vi "Single-Point Tracking.vi"() -> ()   [LabVIEW 2021]
uses:
  <vilib>/myRIO/Instrument Drivers/Onboard IO/I2C/typedefs/I2C User Configuration.ctl
  <vilib>/myRIO/Instrument Drivers/Onboard IO/I2C/typedefs/I2C Transfer Rate.ctl
  <vilib>/myRIO/Instrument Drivers/Onboard IO/I2C/typedefs/I2C Reference.ctl
  <vilib>/myRIO/Common/Instrument Driver Framework/Utilities/typedefs/myRIO Generic Hardware Reference.ctl
  <vilib>/myRIO/Common/Instrument Driver Framework/Utilities/typedefs/Hardware Version Enum.ctl
  <vilib>/myRIO/Common/Instrument Driver Framework/Utilities/typedefs/myRIO v1.0 Reference.ctl
  <vilib>/myRIO/Common/Instrument Driver Framework/Utilities/typedefs/Generic FPGA Reference.ctl
  <vilib>/myRIO/Common/Instrument Driver Framework/myRIO v1.0/I2C/typedefs/I2C Channels Enum.ctl
  <vilib>/myRIO/Instrument Drivers/Onboard IO/I2C/typedefs/I2C Configuration.ctl
  <vilib>/userDefined/High Color/nirio_resource_hc.ctl
  <vilib>/myRIO/Instrument Drivers/Onboard IO/DIO/typedefs/DIO Reference.ctl
  <vilib>/myRIO/Common/Instrument Driver Framework/myRIO v1.0/DIO/typedefs/DIO Channels List.ctl
  <vilib>/myRIO/Common/Instrument Driver Framework/myRIO v1.0/DIO/typedefs/DIO Channels Enum.ctl
  <vilib>/myRIO/Instrument Drivers/Onboard IO/PWM/typedefs/PWM Reference.ctl
  <vilib>/myRIO/Common/Instrument Driver Framework/myRIO v1.0/PWM/typedefs/PWM Channels Enum.ctl
  <vilib>/myRIO/Instrument Drivers/Onboard IO/PWM/typedefs/PWM Configuration.ctl
  <vilib>/myRIO/Common/Instrument Driver Framework/Utilities/vis/Is FPGA Ref Available.vi
  <vilib>/myRIO/Common/Instrument Driver Framework/myRIO v1.0/I2C/vis/myRIO v1.1 Open I2C.vi
  <vilib>/myRIO/Instrument Drivers/Onboard IO/I2C/vis/Configure.vi
  <vilib>/myRIO/Instrument Drivers/Onboard IO/I2C/vis/Write.vi
  <vilib>/myRIO/Common/Instrument Driver Framework/myRIO v1.0/PWM/vis/myRIO v1.1 Open PWM.vi
  <vilib>/myRIO/Instrument Drivers/Onboard IO/PWM/vis/Set Duty Cycle and Frequency.vi
  <vilib>/myRIO/Common/Instrument Driver Framework/myRIO v1.0/DIO/vis/myRIO v1.1 Open DIO.vi
  <vilib>/myRIO/Instrument Drivers/Onboard IO/DIO/vis/Write.vi
  <vilib>/myRIO/Instrument Drivers/Onboard IO/I2C/vis/Write Read.vi
  <vilib>/Analysis/baseanly.llb/Mean (DBL).vi
  <vilib>/myRIO/Common/Instrument Driver Framework/Utilities/vis/Validate Channels.vi
  <vilib>/myRIO/Common/Instrument Driver Framework/myRIO v1.0/I2C/vis/myRIO v1.0 Reserve I2C.vi
  <vilib>/myRIO/Common/Instrument Driver Framework/myRIO v1.0/PWM/vis/myRIO v1.0 Reserve PWM.vi
  <vilib>/myRIO/Common/Instrument Driver Framework/myRIO v1.0/DIO/vis/myRIO v1.0 Reserve DIO.vi
  <vilib>/myRIO/Common/Instrument Driver Framework/myRIO v1.0/UART/vis/myRIO v1.0 Close UART.vi
  <vilib>/myRIO/Common/Instrument Driver Framework/myRIO v1.0/I2C/vis/myRIO v1.0 Build MUX Configuration I2C.vi
  <vilib>/myRIO/Common/Instrument Driver Framework/myRIO v1.0/Resource Manager/vis/myRIO v1.0 Reserve Channel List.vi
  <vilib>/myRIO/Common/Instrument Driver Framework/myRIO v1.0/PWM/vis/myRIO v1.0 Build MUX Configuration PWM.vi
  <vilib>/myRIO/Common/Instrument Driver Framework/myRIO v1.0/DIO/vis/myRIO v1.0 Build MUX Configuration DIO.vi
  <vilib>/myRIO/Common/Instrument Driver Framework/myRIO v1.0/Resource Manager/vis/myRIO v1.0 Create Configuration List.vi
  <vilib>/myRIO/Common/Instrument Driver Framework/myRIO v1.0/Resource Manager/vis/myRIO v1.0 Reserve Channel.vi
  <vilib>/myRIO/Common/Instrument Driver Framework/myRIO v1.0/Resource Manager/vis/myRIO v1.0 Unreserve Channel.vi
  <vilib>/myRIO/Common/Instrument Driver Framework/myRIO v1.0/Resource Manager/vis/myRIO v1.0 Build Mutex Name.vi
  <vilib>/Utility/VariantDataType/GetNumericInfo.vi
  <vilib>/Utility/error.llb/Error Cluster From Error Code.vi
  <vilib>/myRIO/Common/Instrument Driver Framework/myRIO v1.0/myRIO v1.1 Open.vi
  <vilib>/myRIO/Common/Instrument Driver Framework/Utilities/vis/IO Manager.vi
  <vilib>/myRIO/Common/Instrument Driver Framework/Utilities/vis/Configuration Manager.vi
  <vilib>/myRIO/Common/Instrument Driver Framework/myRIO v1.0/Resource Manager/vis/myRIO v1.0 Configure IO.vi
  <vilib>/myRIO/Common/Instrument Driver Framework/myRIO v1.0/myRIO v1.0 Close.vi
  <vilib>/myRIO/Common/Instrument Driver Framework/myRIO v1.0/I2C/vis/myRIO v1.0 Configure I2C.vi
  <vilib>/myRIO/Common/Instrument Driver Framework/myRIO v1.0/I2C/vis/myRIO v1.0 Write I2C.vi
  <vilib>/myRIO/Common/Instrument Driver Framework/myRIO v1.0/DIO/vis/myRIO v1.0 Write DIO.vi
  <vilib>/myRIO/Common/Instrument Driver Framework/myRIO v1.0/PWM/vis/myRIO v1.0 Write PWM.vi
  <vilib>/myRIO/Common/Instrument Driver Framework/myRIO v1.0/I2C/vis/myRIO v1.0 Read I2C.vi
  <vilib>/myRIO/Common/Instrument Driver Framework/Utilities/vis/FPGA Ref Manager.vi
  <vilib>/myRIO/Common/Instrument Driver Framework/myRIO v1.0/myRIO v1.0 Reset FPGA.vi
  <vilib>/myRIO/Common/Instrument Driver Framework/myRIO v1.0/IRQ/vis/myRIO v1.0 IRQ Info FGV.vi
  <vilib>/myRIO/Common/Instrument Driver Framework/myRIO v1.0/IRQ/vis/myRIO v1.0 Timer IRQ Info FGV.vi
  <vilib>/myRIO/Common/Instrument Driver Framework/myRIO v1.0/IRQ/vis/myRIO v1.0 ISR Agent.vi
  <vilib>/myRIO/Instrument Drivers/Utilities/vis/Reset Index.vi
  <vilib>/myRIO/Common/Instrument Driver Framework/myRIO v1.0/Resource Manager/vis/myRIO v1.0 Block Write Resource Manager.vi
  <vilib>/myRIO/Express VI/Onboard IO/I2C/I2C Express VI.xnode
  <vilib>/myRIO/Instrument Drivers/Onboard IO/I2C/vis/myRIO I2C Open.xnode
  <vilib>/myRIO/Express VI/Onboard IO/DO/DO Express VI.xnode
  <vilib>/myRIO/Instrument Drivers/Onboard IO/DIO/vis/myRIO DIO Open.xnode
  <vilib>/myRIO/Express VI/Onboard IO/PWM/PWM Express VI.xnode
  <vilib>/myRIO/Instrument Drivers/Onboard IO/PWM/vis/myRIO PWM Open.xnode
  <vilib>/myRIO/Instrument Drivers/Onboard IO/I2C/I2C.lvlib
  <vilib>/Analysis/NI_AALBase.lvlib
  <vilib>/ptbypt/NI_PtbyPt.lvlib
  <vilib>/myRIO/Instrument Drivers/Onboard IO/PWM/PWM.lvlib
  <vilib>/myRIO/Instrument Drivers/Onboard IO/DIO/DIO.lvlib
  <vilib>/myRIO/Instrument Drivers/Utilities/Utilities.lvlib
panel:
  out "path5":cluster{dbl[], dbl[]}(graph)
  out "distance":dbl
  out "Yaw target":dbl
  out "Yt":dbl
  out "Xt":dbl
  in  "Yg":dbl
  in  "Xg":dbl
  in  "P-gain":dbl
  out "Error":cluster{dbl[], dbl[]}(graph)
  out "Yaw error":dbl
  out "Command/Gauge":cluster{dbl[], dbl[]}[](graph)
  out "angular degree":dbl format="%0.2f"
  out "Velocity duty cycle":dbl(slide) scale=0.0..10.0
  out "Turn duty cycle":dbl(slide) scale=0.0..10.0
  in  "start":bool
  in  "remote":bool
  out "Guage":dbl(knob) scale=0.0..360.0
  out "GZ":dbl format="%0.2f"
  in  "G 歸零":bool
  out "correct GZ":dbl format="%0.2f"
  in  "G 校正":bool
  in  "stop":bool
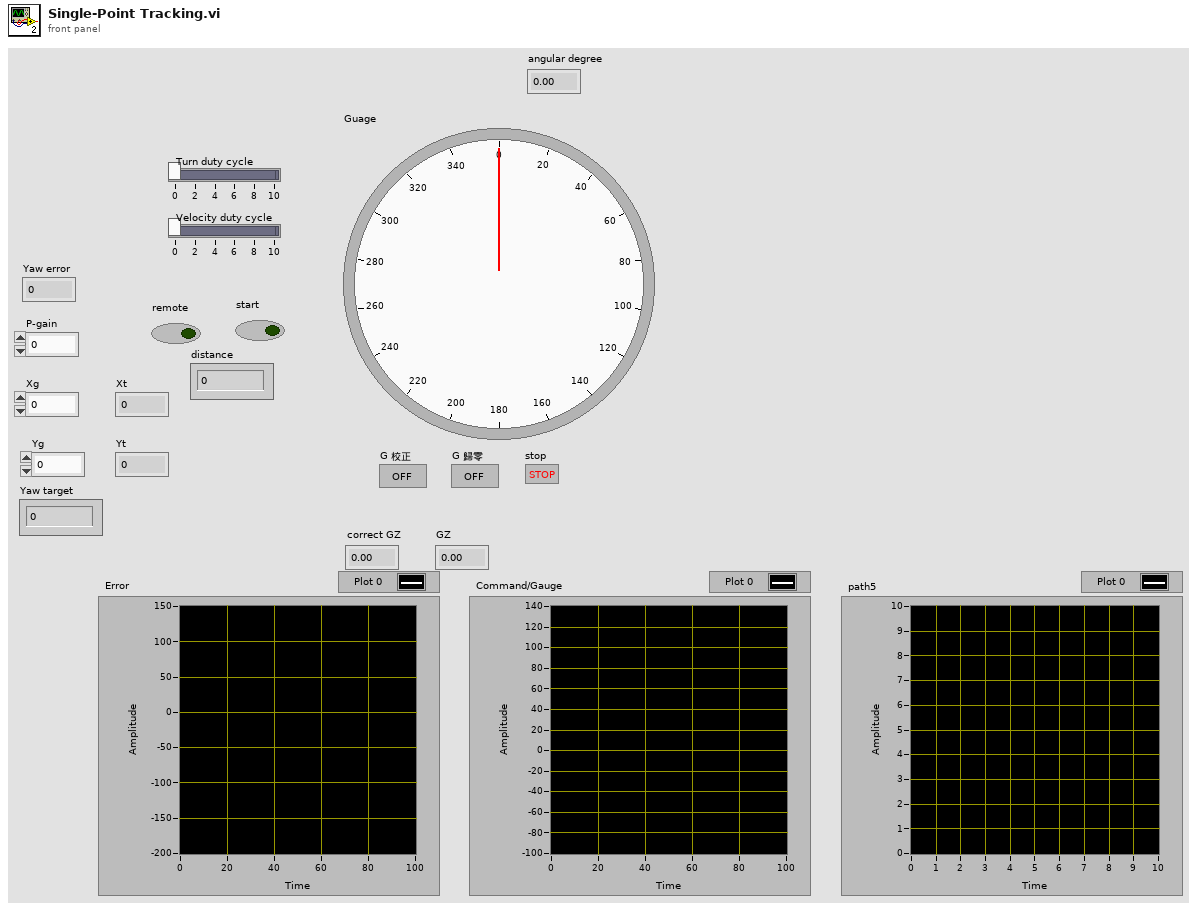
[diagram p1: front panel]
types:
  T1 = typedef "I2C.lvlib/I2C Reference.ctl" = cluster{"myRIO Reference":T2, "I2C Channels Enum":T6, "I2C Configuration":T7}
  T2 = typedef "myRIO Generic Hardware Reference.ctl" = cluster{"myRIO Model":T3, "myRIO Hardware Reference":T4}
  T3 = typedef "Hardware Version Enum.ctl" = enum16{"Unknown", "myRIO-1900", "myRIO-1950", "roboRIO", "NI ELVIS RIO CM", "ELVIS III"}
  T4 = typedef "myRIO v1.0 Reference.ctl" = cluster{"Generic FPGA Reference":T5, "Allow multiple opens":bool}
  T5 = typedef "Generic FPGA Reference.ctl" = refnum<k20>
  T6 = typedef "I2C Channels Enum.ctl" = enum16{"Not Connected", "A/I2C", "B/I2C", "I2C/I2C"}
  T7 = typedef "I2C.lvlib/I2C Configuration.ctl" = cluster{"I2C Transfer Rate":T8}
  T8 = typedef "I2C.lvlib/I2C Transfer Rate.ctl" = enum16{"Standard mode (100 kbps)", "Fast mode (400 kbps)"}
  T9 = typedef "I2C.lvlib/I2C User Configuration.ctl" = cluster{"I2C Transfer Rate":T8}
  T10 = typedef "nirio_resource_hc.ctl" = tag
  T11 = typedef "DIO.lvlib/DIO Reference.ctl" = cluster{"myRIO Reference":T2, "DIO Channels List":T12}
  T12 = typedef "DIO Channels List.ctl" = T13[]
  T13 = typedef "DIO Channels Enum.ctl" = enum16{"Not Connected", "C/DIO0", "C/DIO1", "C/DIO2", "C/DIO3", "C/DIO4", "C/DIO5", "C/DIO6", "C/DIO7", "A/DIO0", "A/DIO1", "A/DIO2", "A/DIO3", "A/DIO4", "A/DIO5", "A/DIO6", "A/DIO7", "A/DIO8", "A/DIO9", "A/DIO10", "A/DIO11", "A/DIO12", "A/DIO13", "A/DIO14", "A/DIO15", "A/DIO16", "A/DIO17", "A/DIO18", "A/DIO19", "B/DIO0", "B/DIO1", "B/DIO2", "B/DIO3", "B/DIO4", "B/DIO5", "B/DIO6", "B/DIO7", "B/DIO8", "B/DIO9", "B/DIO10", "B/DIO11", "B/DIO12", "B/DIO13", "B/DIO14", "B/DIO15", "B/DIO16", "B/DIO17", "B/DIO18", "B/DIO19", "LED0", "LED1", "LED2", "LED3", "Button0", "DIO/DIO0", "DIO/DIO1", "DIO/DIO2", "DIO/DIO3", "DIO/DIO4", "DIO/DIO5", "DIO/DIO6", "DIO/DIO7", "DIO/DIO8", "DIO/DIO9", "SPI/CS0", "SPI/CS1", "SPI/CS2", "SPI/CS3", "LED RADIO (Green)", "LED RADIO (Red)", "LED COMM (Green)", "LED COMM (Red)", "LED MODE (Green)", "LED MODE (Red)"}
  T14 = typedef "PWM.lvlib/PWM Reference.ctl" = cluster{"myRIO Reference":T2, "PWM Channels Enum":T15, "PWM Configuration":T16}
  T15 = typedef "PWM Channels Enum.ctl" = enum16{"Not Connected", "C/PWM0", "C/PWM1", "A/PWM0", "A/PWM1", "A/PWM2", "A/PWM3", "A/PWM4", "A/PWM5", "A/PWM6", "A/PWM7", "A/PWM8", "A/PWM9", "A/PWM10", "A/PWM11", "A/PWM12", "A/PWM13", "A/PWM14", "A/PWM15", "A/PWM16", "A/PWM17", "A/PWM18", "A/PWM19", "B/PWM0", "B/PWM1", "B/PWM2", "B/PWM3", "B/PWM4", "B/PWM5", "B/PWM6", "B/PWM7", "B/PWM8", "B/PWM9", "B/PWM10", "B/PWM11", "B/PWM12", "B/PWM13", "B/PWM14", "B/PWM15", "B/PWM16", "B/PWM17", "B/PWM18", "B/PWM19", "PWM/PWM0", "PWM/PWM1", "PWM/PWM2", "PWM/PWM3", "PWM/PWM4", "PWM/PWM5", "PWM/PWM6", "PWM/PWM7", "PWM/PWM8", "PWM/PWM9"}
  T16 = typedef "PWM.lvlib/PWM Configuration.ctl" = cluster{"Frequency":dbl, "Duty Cycle":dbl}
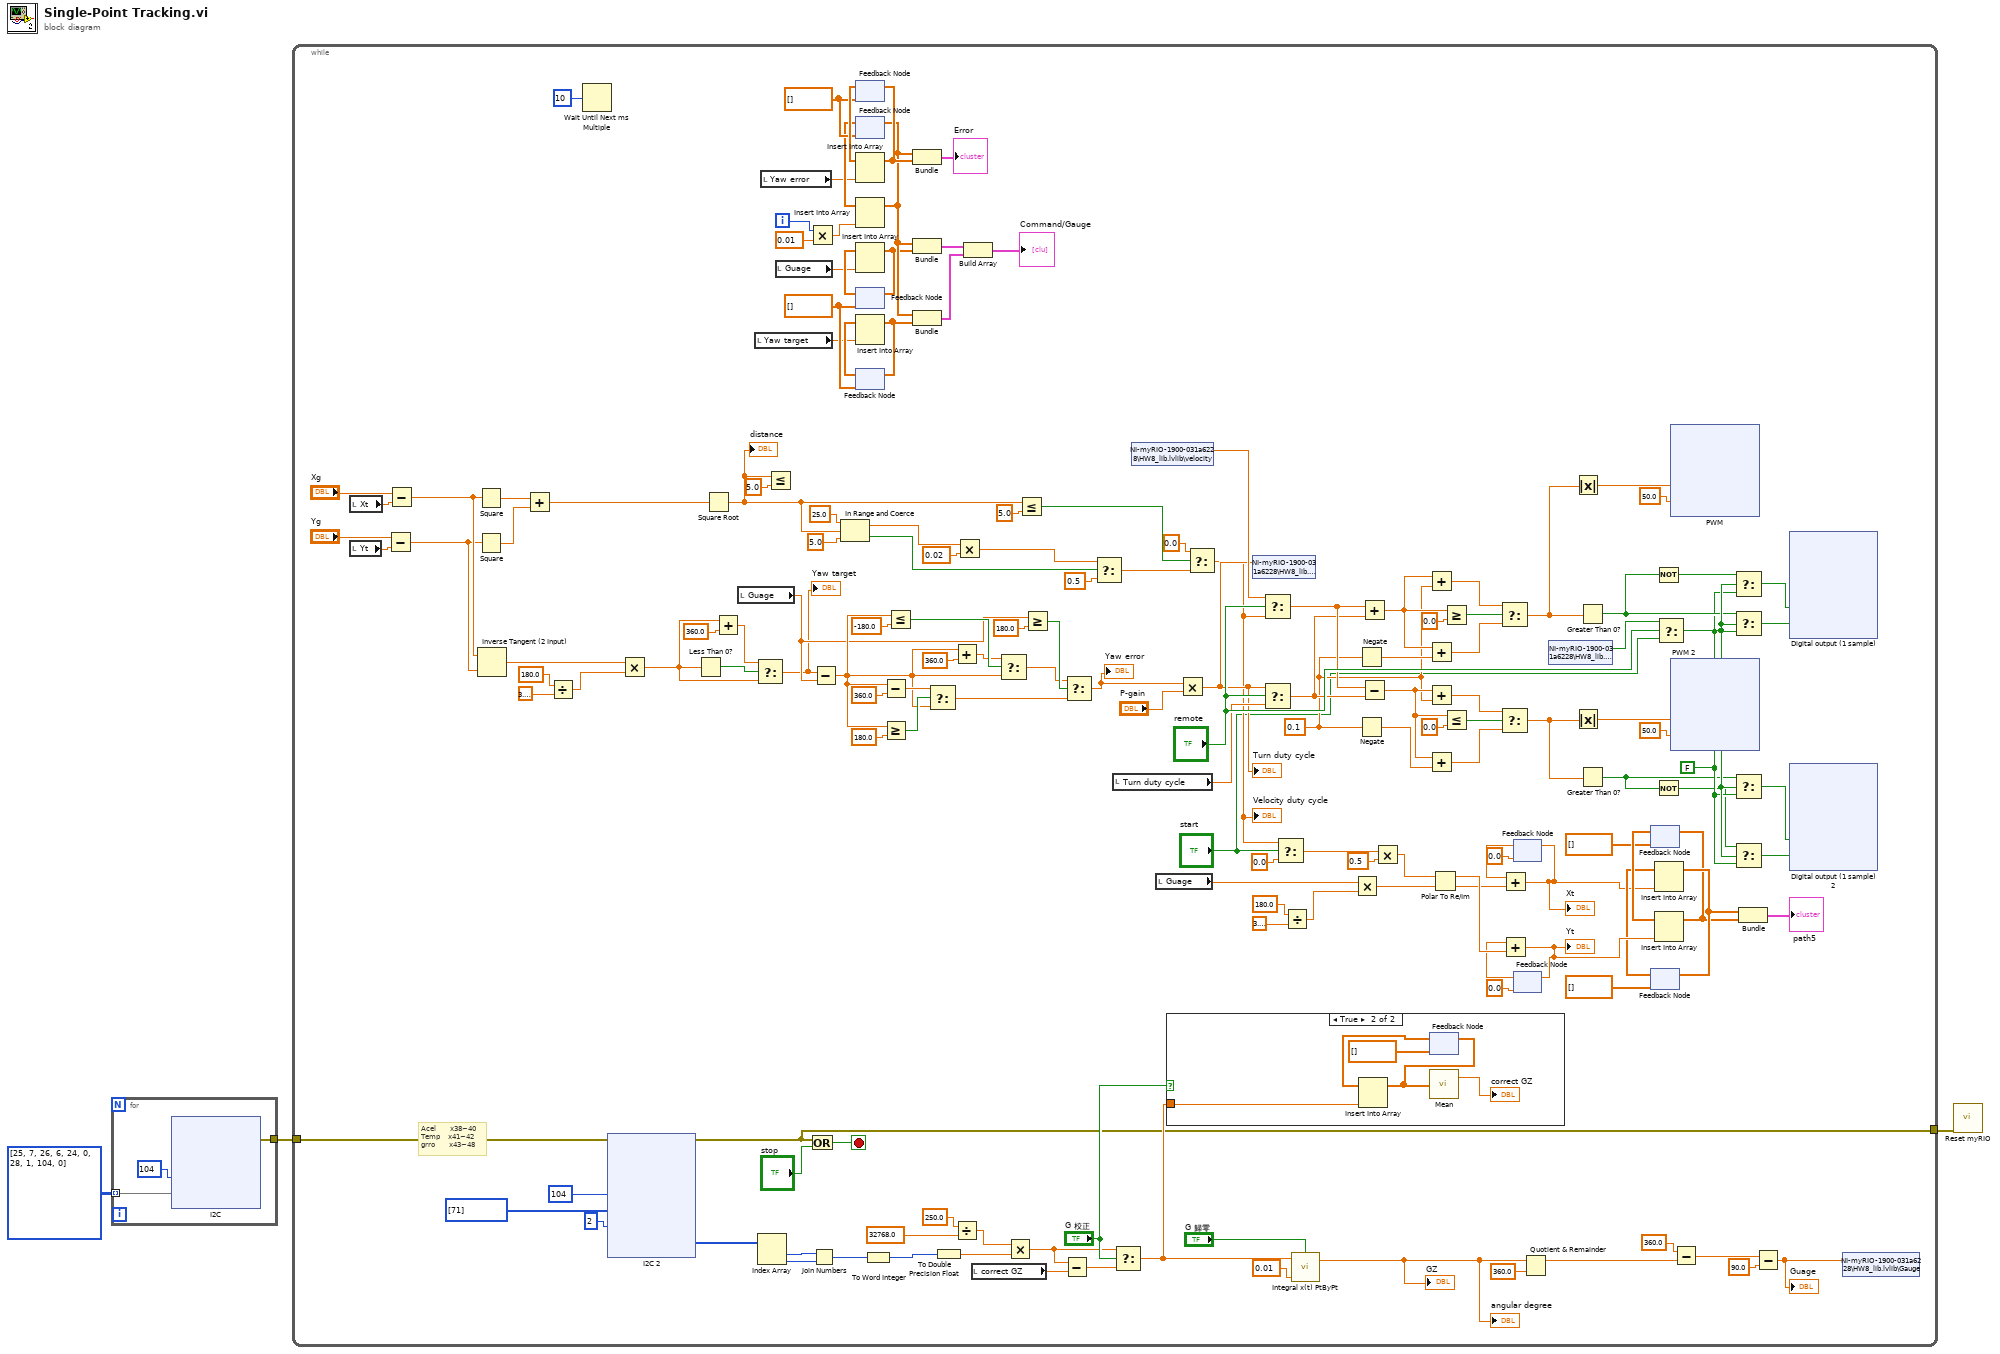
[diagram p0: block diagram]
diagram:
  n1 = for {
    tunnel: u8[][] [[25, 7], [26, 6], [24, 0], [28, 1], [104, 0]] ("Bytes to Write") -> [w6] mode=indexing
    tunnel: [w5] -> w2
    n2 = xnode "I2C"("Slave Address (7-bit)"=u8 104, "Bytes to Write"=w6) -> ("error out"=w5:errorcluster)  [unwired: 1 in]
  }
  n3 = while {
    tunnel: w2 -> [w105]
    tunnel: [w104] -> w1
    i -> [w163]
    stop <- w190 stop-if-true
    w127 = 0.1 ("y")
    w165 = dbl[] []
    w170 = dbl[] []
    w180 = FALSE
    # "Acel       x38~40\nTemp    x41~42\ngrro       x43~48"
    n4 = local read "Xt"() -> (w101:dbl)
    n5 = local read "Yt"() -> (w99:dbl)
    n6 = Subtract(x="Yg", y=w99) -> (x-y=w97:dbl)
    n7 = Subtract(x="Xg", y=w101) -> (x-y=w98:dbl)
    n8 = Square(x=w98) -> (x^2=w96:dbl)
    n9 = Square(x=w97) -> (x^2=w95:dbl)
    n10 = Inverse Tangent (2 Input)(1:w97, 2:w98) -> (0:w93:dbl)
    n11 = Add(x=w96, y=w95) -> (x+y=w94:dbl)
    n12 = Divide(x=180.0, y=3.141592653589793) -> (x/y=w90:dbl)
    n13 = Wait Until Next ms Multiple(millisecond multiple=u32 10) -> ()  [unwired: 1 out]
    n14 = xnode "I2C 2"("Slave Address (7-bit)"=u8 104, "Bytes to Write"=u8[] [71], "Byte Count"=u32 2, "error in (no error)"=w105) -> ("Bytes Read"=w103:u8[], "error out"=w104:errorcluster)
    n15 = Multiply(x=w93, y=w90) -> (x*y=w88:dbl)
    n16 = Less Than 0?(x=w88) -> (x < 0?=w89:bool)
    n17 = Square Root(x=w94) -> (sqrt(x)=w76:dbl)
    "distance" <- w76
    n18 = Add(x=w88, y=360.0) -> (x+y=w86:dbl)
    n19 = local read "Guage"() -> (w109:dbl)
    n20 = local read "Yaw target"() -> (w156:dbl)
    n21 = Select(t=w86, s=w89, f=w88) -> (s? t:f=w85:dbl)
    "Yaw target" <- w85
    n22 = Index Array(array=w103) -> (element #1=w204:u8, element #2=w203:u8)  [unwired: 2 in]
    n23 = local read "Yaw error"() -> (w155:dbl)
    n24 = Less Or Equal?(x=w76, y=5.0) -> ()  [unwired: 1 out]
    n25 = local read "Guage"() -> (w110:dbl)
    n26 = Multiply(x=w163, y=0.01) -> (x*y=w172:dbl)
    n27 = Or(x=w104, y="stop") -> (x .or. y?=w190:bool)
    n28 = Join Numbers(hi=w204, lo=w203) -> ((hi.lo)=w202:u16)
    n29 = Subtract(x=w85, y=w109) -> (x-y=w143:dbl)
    n30 = In Range and Coerce(upper limit=25.0, x=w76, lower limit=5.0) -> (coerced(x)=w81:dbl, In Range?=w79:bool)
    n31 = feedback #1(w170) -> (w171:dbl[])
    n32 = feedback #2(w170) -> (w164:dbl[])
    n33 = Insert Into Array(array=w171, new element=w155) -> (w169:dbl[])  [unwired: 1 in]
    n34 = feedback-in #1(w169) -> ()
    n35 = Insert Into Array(array=w164, new element=w172) -> (w162:dbl[])  [unwired: 1 in]
    n36 = feedback-in #2(w162) -> ()
    n37 = feedback #3(w165) -> (w167:dbl[])
    n38 = Insert Into Array(array=w167, new element=w110) -> (w161:dbl[])  [unwired: 1 in]
    n39 = feedback-in #3(w161) -> ()
    n40 = feedback #4(w165) -> (w166:dbl[])
    n41 = Insert Into Array(array=w166, new element=w156) -> (w160:dbl[])  [unwired: 1 in]
    n42 = feedback-in #4(w160) -> ()
    n43 = To Word Integer(number=w202) -> (16bit integer=w199:i16)
    n44 = Subtract(x=w143, y=360.0) -> (x-y=w144:dbl)
    n45 = Greater Or Equal?(x=w143, y=180.0) -> (x >= y?=w151:bool)
    n46 = Less Or Equal?(x=w143, y=-180.0) -> (x <= y?=w152:bool)
    n47 = Bundle(w162, w169) -> (→"Error":cluster{dbl[], dbl[]})  [unwired: 1 in]
    n48 = Bundle(w162, w161) -> (w159:cluster{dbl[], dbl[]})  [unwired: 1 in]
    n49 = Bundle(w162, w160) -> (w158:cluster{dbl[], dbl[]})  [unwired: 1 in]
    n50 = Select(t=w144, s=w151, f=w143) -> (s? t:f=w145:dbl)
    n51 = To Double Precision Float(number=w199) -> (double precision float=w192:dbl)
    n52 = Add(x=w143, y=360.0) -> (x+y=w142:dbl)
    n53 = Divide(x=250.0, y=32768.0) -> (x/y=w198:dbl)
    n54 = Multiply(x=w81, y=0.02) -> (x*y=w78:dbl)
    n55 = Build Array(w159, w158) -> (→"Command/Gauge":cluster{dbl[], dbl[]}[])
    n56 = local read "correct GZ"() -> (w118:dbl)
    n57 = Select(t=w142, s=w152, f=w143) -> (s? t:f=w146:dbl)
    n58 = Multiply(x=w198, y=w192) -> (x*y=w174:dbl)
    n59 = Less Or Equal?(x=w76, y=5.0) -> (x <= y?=w74:bool)
    n60 = Greater Or Equal?(x=w109, y=180.0) -> (x >= y?=w149:bool)
    n61 = Subtract(x=w174, y=w118) -> (x-y=w191:dbl)
    n62 = Select(t=w146, s=w149, f=w145) -> (s? t:f=w140:dbl)
    "Yaw error" <- w140
    n63 = Select(t=w78, s=w79, f=0.5) -> (s? t:f=w73:dbl)
    n64 = local read "Turn duty cycle"() -> (w139:dbl)
    n65 = Select(t=w174, s="G 校正", f=w191) -> (s? t:f=w175:dbl)
    n66 = shared-variable "NI-myRIO-1900-031a6228\\HW8_lib.lvlib\\velocity"() -> (w120:dbl)  [unwired: 1 in, 1 out]
    n67 = local read "Guage"() -> (w66:dbl)
    n68 = case shown="True" "G 校正" {
      tunnel: w175 -> [_ w387]
      frame False {
      }
      frame True {
        n69 = feedback #5(dbl[] []) -> (w391:dbl[])
        n70 = Insert Into Array(array=w391, new element=w387) -> (w389:dbl[])  [unwired: 1 in]
        n71 = feedback-in #5(w389) -> ()
        n72 = call-poly <vilib>:"Mean.vi"("X"=w389) -> ("mean"=→"correct GZ":dbl)  [unwired: 1 out]
      }
    }
    n73 = Multiply(x=w140, y="P-gain") -> (x*y=w119:dbl)
    "Turn duty cycle" <- w119
    n74 = Select(t=0.0, s=w74, f=w73) -> (s? t:f=w71:dbl)
    "Velocity duty cycle" <- w71
    n75 = shared-variable "NI-myRIO-1900-031a6228\\HW8_lib.lvlib\\turn"(w119) -> ()  [unwired: 1 in, 1 out]
    n76 = Select(t=w120, s="remote", f=w71) -> (s? t:f=w138:dbl)
    n77 = Select(t=w119, s="remote", f=w139) -> (s? t:f=w137:dbl)
    n78 = Select(t=w71, s="start", f=0.0) -> (s? t:f=w68:dbl)
    n79 = Divide(x=180.0, y=3.141592653589793) -> (x/y=w63:dbl)
    n80 = call <vilib>:"Integral x(t) PtByPt.vi"("initialize"="G 歸零", "dt"=0.01, "x"=w175) -> ("integral x(t)"=w196:dbl)  [unwired: 1 in, 1 out]
    "GZ" <- w196
    "angular degree" <- w196
    n81 = Multiply(x=w66, y=w63) -> (x*y=w61:dbl)
    n82 = Negate(x=w127) -> (-x=w132:dbl)
    n83 = Negate(x=w127) -> (-x=w126:dbl)
    n84 = Add(x=w138, y=w137) -> (x+y=w133:dbl)
    n85 = Subtract(x=w138, y=w137) -> (x-y=w129:dbl)
    n86 = Multiply(x=w68, y=0.5) -> (x*y=w62:dbl)
    n87 = Add(x=w133, y=w127) -> (x+y=w130:dbl)
    n88 = Add(x=w133, y=w132) -> (x+y=w131:dbl)
    n89 = Add(x=w129, y=w127) -> (x+y=w128:dbl)
    n90 = Add(x=w129, y=w126) -> (x+y=w125:dbl)
    n91 = Polar To Re/Im(2:w61, 3:w62) -> (0:w54:dbl, 1:w60:dbl)
    n92 = Greater Or Equal?(x=w133, y=0.0) -> (x >= y?=w134:bool)
    n93 = Less Or Equal?(x=w129, y=0.0) -> (x <= y?=w124:bool)
    n94 = Select(t=w130, s=w134, f=w131) -> (s? t:f=w122:dbl)
    n95 = Select(t=w128, s=w124, f=w125) -> (s? t:f=w123:dbl)
    n96 = feedback #6(0.0) -> (w53:dbl)
    n97 = Add(x=w53, y=w54) -> (x+y=w49:dbl)
    "Xt" <- w49
    n98 = feedback-in #6(w49) -> ()
    n99 = feedback #7(0.0) -> (w59:dbl)
    n100 = Add(x=w59, y=w60) -> (x+y=w57:dbl)
    "Yt" <- w57
    n101 = feedback-in #7(w57) -> ()
    n102 = Quotient & Remainder(x=w196, y=360.0) -> (x-y*floor(x/y)=w194:dbl)  [unwired: 1 out]
    n103 = shared-variable "NI-myRIO-1900-031a6228\\HW8_lib.lvlib\\start"() -> (w121:bool)  [unwired: 1 in, 1 out]
    n104 = Absolute Value(x=w122) -> (abs(x)=w188:dbl)
    n105 = Absolute Value(x=w123) -> (abs(x)=w187:dbl)
    n106 = Greater Than 0?(x=w122) -> (x > 0?=w181:bool)
    n107 = Greater Than 0?(x=w123) -> (x > 0?=w178:bool)
    n108 = feedback #8(dbl[] []) -> (w56:dbl[])
    n109 = feedback #9(dbl[] []) -> (w51:dbl[])
    n110 = Not(x=w181) -> (.not. x?=w184:bool)
    n111 = Not(x=w178) -> (.not. x?=w179:bool)
    n112 = Insert Into Array(array=w51, new element=w49) -> (w48:dbl[])  [unwired: 1 in]
    n113 = feedback-in #9(w48) -> ()
    n114 = Insert Into Array(array=w56, new element=w57) -> (w47:dbl[])  [unwired: 1 in]
    n115 = feedback-in #8(w47) -> ()
    n116 = Select(t=w121, s="remote", f="start") -> (s? t:f=w182:bool)
    n117 = xnode "PWM"("Duty Cycle"=w188, "Frequency [Hz]"=50.0) -> ()  [unwired: 1 in, 1 out]
    n118 = xnode "PWM 2"("Duty Cycle"=w187, "Frequency [Hz]"=50.0) -> ()  [unwired: 1 in, 1 out]
    n119 = Subtract(x=360.0, y=w194) -> (x-y=w112:dbl)
    n120 = Select(t=w184, s=w182, f=w180) -> (s? t:f=w117:bool)
    n121 = Select(t=w181, s=w182, f=w180) -> (s? t:f=w116:bool)
    n122 = Select(t=w178, s=w182, f=w180) -> (s? t:f=w115:bool)
    n123 = Select(t=w179, s=w182, f=w180) -> (s? t:f=w114:bool)
    n124 = Bundle(w48, w47) -> (→"path5":cluster{dbl[], dbl[]})  [unwired: 1 in]
    n125 = Subtract(x=w112, y=90.0) -> (x-y=w111:dbl)
    "Guage" <- w111
    n126 = xnode "Digital output (1 sample)"("C/DIO2 (DIO2)"=w117, "C/DIO1 (DIO1)"=w116) -> ()  [unwired: 1 in, 1 out]
    n127 = xnode "Digital output (1 sample) 2"("C/DIO6 (DIO6)"=w115, "C/DIO5 (DIO5)"=w114) -> ()  [unwired: 1 in, 1 out]
    n128 = shared-variable "NI-myRIO-1900-031a6228\\HW8_lib.lvlib\\Gauge"(w111) -> ()  [unwired: 1 in, 1 out]
  }
  n129 = call <vilib>:"Reset myRIO.vi"("error in (no error)"=w1) -> ()  [unwired: 10 in, 1 out]
